vi "Logging Module.vi"(6 "Logging process enabled":bool, 8 "Data Queue error in":errorcluster, 11 "Queues Cluster":T1) -> (0 "error out":errorcluster)   [LabVIEW 2017]
doc: "The message loop subVI to handle messages pertaining to logging data."
uses:
  User Interface/Queue/Message Queue/Typedefs/All Message Queues.ctl
  User Interface/Queue/Message Queue/Typedefs/Message Cluster.ctl
  Typedefs/Logging queue element.ctl
  Typedefs/Imaging Protocols enum.ctl
  Typedefs/Frame Size.ctl
  Typedefs/Acquired points count.ctl
  Typedefs/Read Write Enum.ctl
  Global Variables/General Globals.vi
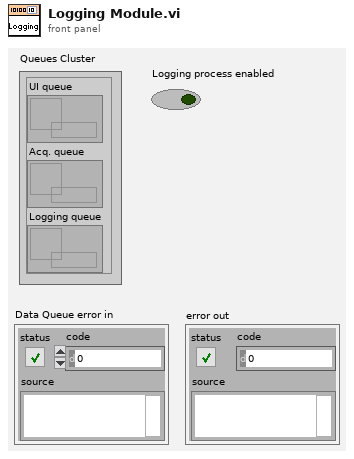
[diagram p1: front panel]
types:
  T1 = typedef "All Message Queues.ctl" = cluster{"UI queue":refnum<queue>, "Acq. queue":refnum<queue>, "Logging queue":refnum<queue>}
  T2 = typedef "Read Write Enum.ctl" = enum16{"Read", "Write"}
  T3 = typedef "ROI File Generator Queue Ref.ctl" = refnum<queue>
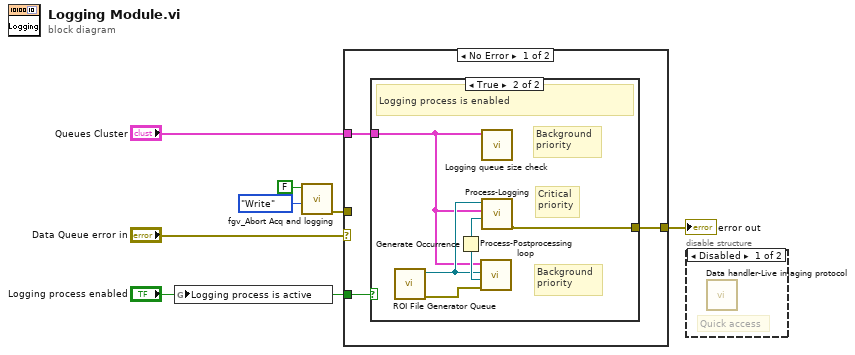
[diagram p0: block diagram]
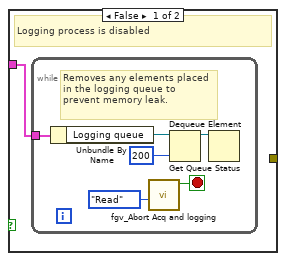
[diagram p3: hidden frame]
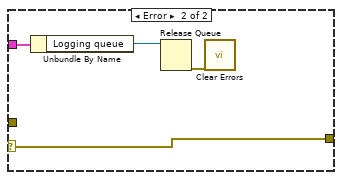
[diagram p4: hidden frame]
diagram:
  n1 = global write "General Globals.vi" "Logging process is active"("Logging process enabled") -> ()
  n2 = call "fgv_Abort Acq and logging.vi"("Function"=Read_Write_Enum."Write", "Live Imaging?"=FALSE) -> ("error out"=w2:errorcluster)  [unwired: 8 in, 1 out]
  n3 = case shown="No Error" "Data Queue error in" {
    selector: "Data Queue error in" -> [_ w23]
    tunnel: "Queues Cluster" -> [w10 w25]
    tunnel: "Logging process enabled" -> [w9 _]
    tunnel: [w8 w23] -> w5
    tunnel: w2 -> [_ _]
    frame No Error {
      n4 = case shown="True" w9 {
        tunnel: w10 -> [w11 w18]
        tunnel: [_ w22] -> w8
        frame False {
          # "Logging process is disabled"
          n5 = while {
            tunnel: w11 -> [w13]
            stop <- w14 stop-if-true
            # "Removes any elements placed in the logging queue to prevent memory leak."
            n6 = Unbundle By Name(w13) -> ("Logging queue"=w12:refnum<queue>)
            n7 = call "fgv_Abort Acq and logging.vi"("Function"=Read_Write_Enum."Read") -> ("Abort acquisition"=w14:bool)  [unwired: 9 in, 1 out]
            n8 = Dequeue Element(queue=w12, timeout in ms (-1)=200) -> (queue out=w16:refnum<queue>)  [unwired: 1 in, 3 out]
            n9 = Get Queue Status(queue=w16) -> ()  [unwired: 2 in, 8 out]
          }
        }
        frame True {
          # "Background\npriority"
          # "Background\npriority"
          # "Critical \npriority"
          # "Logging process is enabled"
          n10 = call "ROI File Generator Queue.vi"() -> ("error out"=w21:errorcluster, "Data-gen queue"=w19:T3)  [unwired: 10 in]
          n11 = Generate Occurrence() -> (w20:refnum<k4>)
          n12 = call "Process-Postprocessing loop.vi"("error"=w21, "occurrence"=w20, "Data-gen queue"=w19, "Queues Cluster"=w18) -> ()  [unwired: 8 in]
          n13 = call "Logging queue size check.vi"("Queues refs"=w18) -> ()  [unwired: 9 in, 2 out]
          n14 = call "Process-Logging.vi"("Wait on post-processing"=w20, "Queues Cluster"=w18, "Data-gen queue"=w19) -> ("error out"=w22:errorcluster)  [unwired: 8 in]
        }
      }
    }
    frame Error {
      n15 = Unbundle By Name(w25) -> ("Logging queue"=w24:refnum<queue>)
      n16 = Release Queue(queue=w24) -> (error out=w26:errorcluster)  [unwired: 2 in, 2 out]
      n17 = call <vilib>:"Clear Errors.vi"("error in (no error)"=w26) -> ()  [unwired: 5 in, 2 out]
    }
  }
  "error out" <- w5
  n18 = disable-structure shown="Disabled" {
    frame Disabled {
      # "Quick access"
      n19 = call "Data handler-Live imaging protocol.vi"() -> ()  [unwired: 11 in, 1 out]
    }
    frame Enabled {
    }
  }
